vi "test Counter Data Plugin Initialize Invalid Object.vi"(8 "error in (no error)":errorcluster, 11 "TestCase in":refnum<class "Data Engine Unit Tests.lvclass">) -> (0 "error out":errorcluster, 3 "TestCase out":refnum<class "Data Engine Unit Tests.lvclass">)   [LabVIEW 2017, in "Data Engine Unit Tests.lvclass"]
uses:
  Data Engine Unit Tests.lvclass
  Source/Counter Data Plugin/Counter Data Plugin.lvclass
  <vilib>/addons/_JKI Toolkits/VI Tester/TestCase.llb/TestCase.lvclass
  C:/Program Files/National Instruments/LabVIEW 2017/vi.lib/addons/_JKI Toolkits/VI Tester/TestCase.llb/TestCase.lvclass
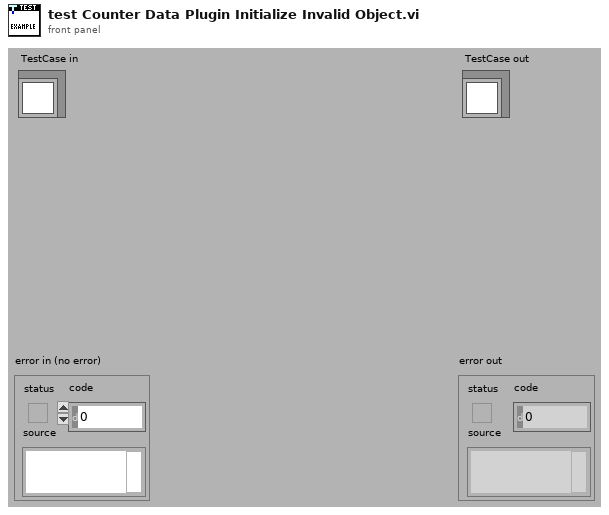
[diagram p1: front panel]
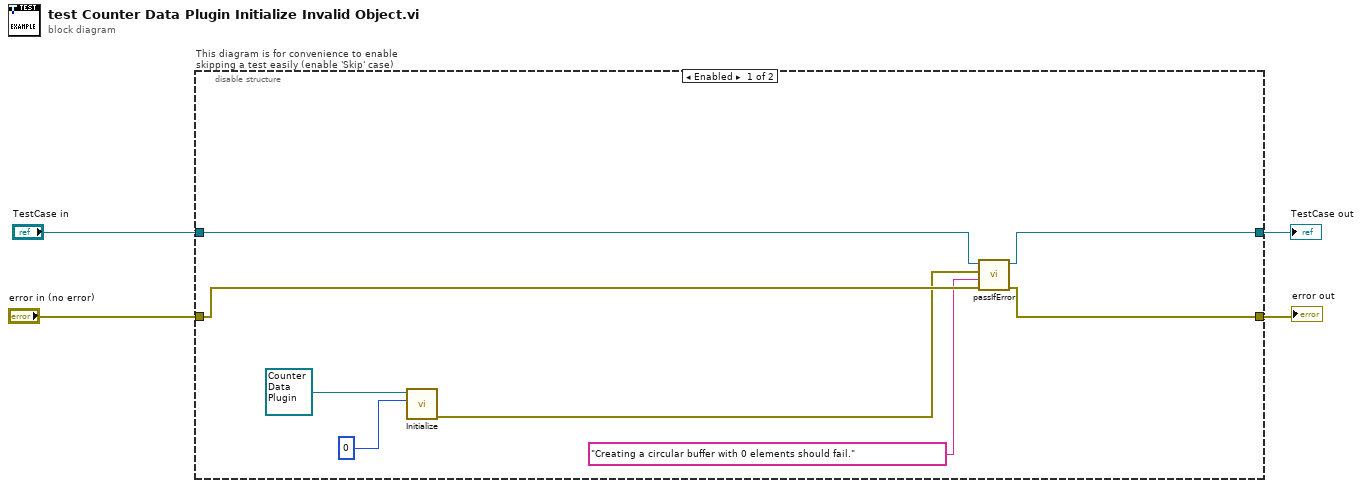
[diagram p0: block diagram]
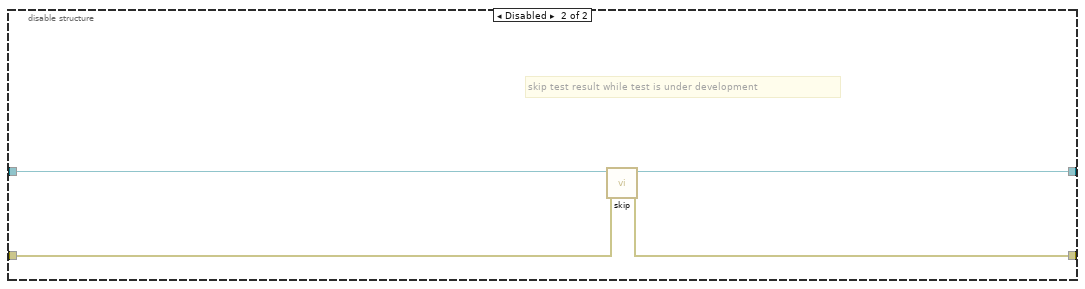
[diagram p2: hidden frame]
diagram:
  n1 = disable-structure "This diagram is for convenience to enable skipping a test easily (enable 'Skip' case)" shown="Enabled" {
    disable-tunnel: "TestCase in" -> [w12 w16]
    disable-tunnel: [w11 w14] -> w1
    disable-tunnel: [w10 w15] -> w3
    disable-tunnel: "error in (no error)" -> [w7 w13]
    frame Enabled {
      n2 = call-dynamic "Initialize.vi"("Circular Buffer Size"=0, "Data Plugin in"=refnum<class "Counter Data Plugin.lvclass"> refnum ("Data Engine.lvlib:Counter Data Plugin.lvclass")) -> ("error out"=w6:errorcluster)  [unwired: 8 in, 1 out]
      n3 = call-dynamic "passIfError.vi"("error in (no error)"=w7, "task (\"\")"="Creating a circular buffer with 0 elements should fail." ("task (\"\")"), "error"=w6, "TestCase in"=w12) -> ("error out"=w10:errorcluster, "TestCase out"=w11:refnum<class "Data Engine Unit Tests.lvclass">)  [unwired: 6 in]
    }
    frame Disabled {
      # "skip test result while test is under development"
      n4 = call <vilib>:"skip.vi"("error in (no error)"=w13, "TestCase in"=w16) -> ("error out"=w15:errorcluster, "TestCase out"=w14:refnum<class "Data Engine Unit Tests.lvclass">)  [unwired: 8 in]
    }
  }
  "error out" <- w3
  "TestCase out" <- w1
